vi "Exponential Fit Coefficients.vi"(0 "Y":dbl[](array[numeric]), 5 "X":dbl[](array[numeric]), 7 "Weight":dbl[](array[numeric]), 9 "tolerance":dbl=0.0001 format="%#_3g", 11 "method":T1 items=["Least Square", "Least Absolute Residual", "Bisquare"], 12 "refine?":bool) -> (4 "amplitude":dbl, 6 "damping":dbl, 15 "error":i32)   [LabVIEW 2018, in "NI_AALPro.lvlib"]
doc: "Returns the <B>amplitude</B> and <B>damping</B> of the exponential fit for a data set (<B>X</B>, <B>Y</B>) using the Least Square, Least Absolute Residual, or Bisquare method."
uses:
  <vilib>/Analysis/NI_AALPro.lvlib
  <vilib>/Analysis/6fits.llb/Curve Fitting Criteria.ctl
panel:
  # "Exponential Fit Coefficients"
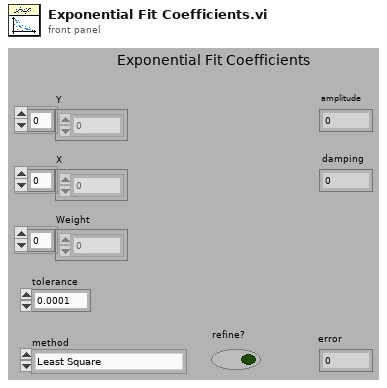
[diagram p1: front panel]
types:
  T1 = typedef "NI_AALPro.lvlib/Curve Fitting Criteria.ctl" = u16
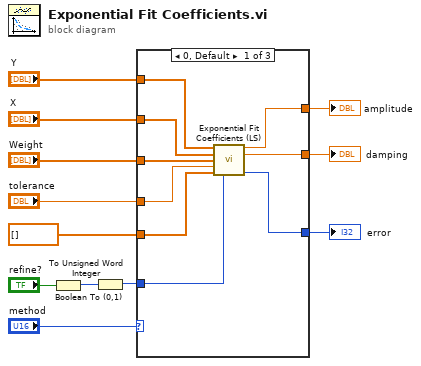
[diagram p0: block diagram]
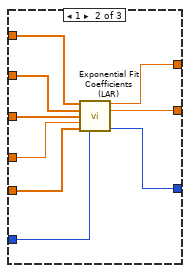
[diagram p2: hidden frame]
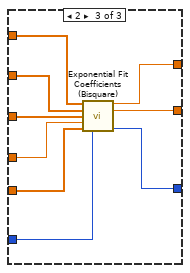
[diagram p3: hidden frame]
diagram:
  n1 = Boolean To (0,1)(Boolean="refine?") -> (0, 1=w1:i16)
  n2 = To Unsigned Word Integer(number=w1) -> (unsigned 16bit integer=w2:u16)
  n3 = case shown="0, Default" "method" {
    tunnel: "Y" -> [w21 w30 w39]
    tunnel: "X" -> [w20 w29 w38]
    tunnel: "Weight" -> [w19 w28 w37]
    tunnel: "tolerance" -> [w18 w27 w36]
    tunnel: dbl[] [] ("Initial Coefficients") -> [w17 w26 w35]
    tunnel: w2 -> [w16 w25 w34]
    tunnel: [w15 w23 w32] -> w6
    tunnel: [w14 w24 w33] -> w5
    tunnel: [w13 w22 w31] -> w4
    frame 0, Default {
      n4 = call "Exponential Fit Coefficients (LS).vi"("Y"=w21, "X"=w20, "Weight"=w19, "tolerance"=w18, "Initial Coefficients"=w17, "algorithm"=w16) -> ("amplitude"=w14:dbl, "damping"=w15:dbl, "error"=w13:i32)  [unwired: 7 out]
    }
    frame 1 {
      n5 = call "Exponential Fit Coefficients (LAR).vi"("Y"=w30, "X"=w29, "Weight"=w28, "tolerance"=w27, "Initial Coefficients"=w26, "algorithm"=w25) -> ("amplitude"=w24:dbl, "damping"=w23:dbl, "error"=w22:i32)  [unwired: 7 out]
    }
    frame 2 {
      n6 = call "Exponential Fit Coefficients (Bisquare).vi"("Y"=w39, "X"=w38, "Weight"=w37, "tolerance"=w36, "Initial Coefficients"=w35, "algorithm"=w34) -> ("amplitude"=w33:dbl, "damping"=w32:dbl, "error"=w31:i32)  [unwired: 7 out]
    }
  }
  "amplitude" <- w5
  "damping" <- w6
  "error" <- w4
